vi "Analysiswangtest.vi"(8 "error in (no error)":errorcluster, 11 "ADC array":i32[][](array[numeric])) -> (0 "error out":errorcluster, 3 "Results":T1)   [LabVIEW 2014]
uses:
  <vilib>/Analysis/NI_AALBase.lvlib
panel:
  in  "Results 2":T1
  # "CH0"
  # "CH1"
  # "CH2"
  # "CH3"
  # "CH4"
  # "CH5"
  # "CH6"
  # "CH7"
  # "CH0"
  # "CH1"
  # "CH2"
  # "CH3"
  # "CH4"
  # "CH5"
  # "CH6"
  # "CH7"
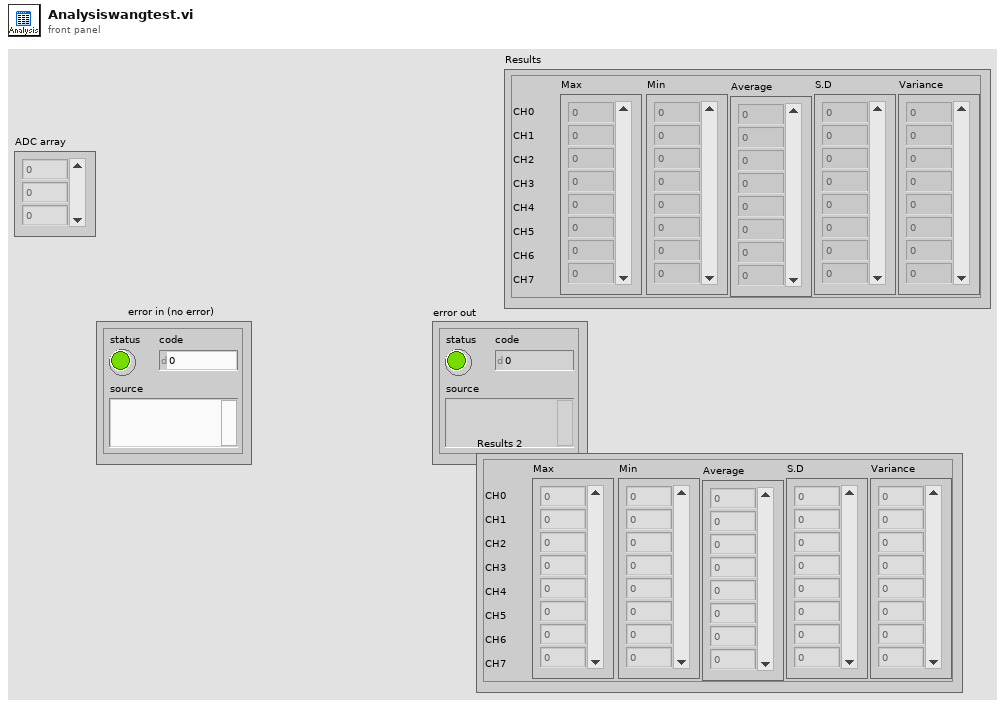
[diagram p1: front panel]
types:
  T1 = cluster{"Max":i32[], "Min":i32[], "Average":dbl[], "S.D":dbl[], "Variance":dbl[]}
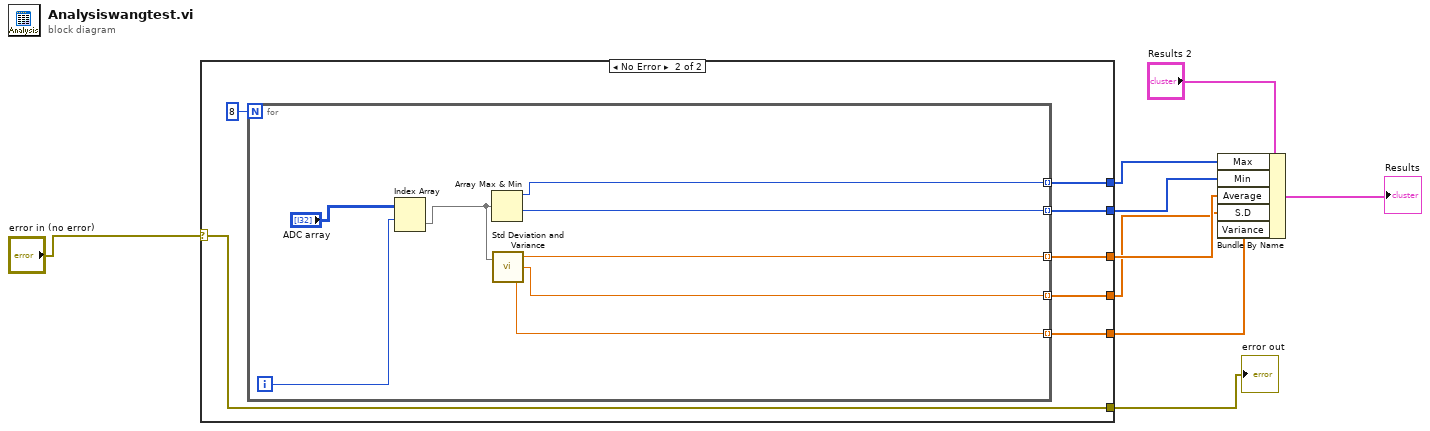
[diagram p0: block diagram]
diagram:
  n1 = case shown="No Error" "error in (no error)" {
    selector: "error in (no error)" -> [w10 w11]
    tunnel: [_ w16] -> w6
    tunnel: [_ w15] -> w5
    tunnel: [_ w14] -> w4
    tunnel: [_ w13] -> w3
    tunnel: [_ w12] -> w2
    tunnel: [w10 w11] -> w8
    frame Error {
    }
    frame No Error {
      n2 = for {
        N: 8 -> [_]
        tunnel: [w23] -> w16 mode=indexing
        tunnel: [w21] -> w15 mode=indexing
        tunnel: [w20] -> w14 mode=indexing
        tunnel: [w19] -> w13 mode=indexing
        tunnel: [w18] -> w12 mode=indexing
        i -> [w24]
        n3 = Index Array(array="ADC array", index (row)=w24) -> (element=w22:i32[])  [unwired: 1 in]
        n4 = Array Max & Min(array=w22) -> (max value=w23:i32, min value=w21:i32)  [unwired: 2 out]
        n5 = call <vilib>:"Std Deviation and Variance.vi"("X"=w22) -> ("mean"=w20:dbl, "standard deviation"=w19:dbl, "variance"=w18:dbl)  [unwired: 1 in]
      }
    }
  }
  "error out" <- w8
  n6 = Bundle By Name(cluster="Results 2", "Max"=w6, "Min"=w5, "Average"=w4, "S.D"=w3, "Variance"=w2) -> (→"Results":T1)
